vi "Calculate_duty_cycle.vi"(10 "Odour bottles in":T2(array[cluster])=[[{"Mixture components"=[{"Name"="MINERAL OIL", "CID"=0, "Volatility"=0.0}], "Name"="B1 (Bl)", "VPs"="0.0E+0", "Proportion"=[{"Numeric"=100.0}], "Selected"=FALSE, "Counter"=TRUE}, {"Mixture components"=[{"Name"="Methyl benzoate", "CID"=8103, "Volatility"=0.38}, {"Name"="Menthone", "CID"=8063, "Volatility"=0.28}], "Name"="B3 (ME2)", "VPs"="3.3E-1 ± 21%", "Proportion"=[{"Numeric"=50.0}, {"Numeric"=50.0}], "Selected"=TRUE, "Counter"=FALSE}, {"Mixture components"=[{"Name"="Decanol", "CID"=460, "Volatility"=0.00851}], "Name"="B5 (C4f)", "VPs"="8.5E-3", "Proportion"=[{"Numeric"=100.0}], "Selected"=FALSE, "Counter"=FALSE}, {"Mixture components"=[{"Name"="Acetophenone", "CID"=8174, "Volatility"=0.45}, {"Name"="Fenchone", "CID"=8635, "Volatility"=0.82}], "Name"="B7 (ME1)", "VPs"="6.4E-1 ± 41%", "Proportion"=[{"Numeric"=50.0}, {"Numeric"=50.0}], "Selected"=FALSE, "Counter"=FALSE}], [{"Mixture components"=[{"Name"="MINERAL OIL", "CID"=0, "Volatility"=0.0}], "Name"="B2 (Bl)", "VPs"="0.0E+0", "Proportion"=[{"Numeric"=100.0}], "Selected"=FALSE, "Counter"=TRUE}, {"Mixture components"=[{"Name"="Octanol", "CID"=7439, "Volatility"=0.0794}], "Name"="B4 (C4cA)", "VPs"="7.9E-2", "Proportion"=[{"Numeric"=100.0}], "Selected"=FALSE, "Counter"=FALSE}, {"Mixture components"=[{"Name"="MINERAL OIL", "CID"=0, "Volatility"=0.0}], "Name"="B6 (Bl)", "VPs"="0.0E+0", "Proportion"=[{"Numeric"=100.0}], "Selected"=FALSE, "Counter"=FALSE}, {"Mixture components"=[{"Name"="Heptanoic acid ", "CID"=957, "Volatility"=0.0107}], "Name"="B8 (C3cA)", "VPs"="1.1E-2", "Proportion"=[{"Numeric"=100.0}], "Selected"=FALSE, "Counter"=FALSE}], [{"Mixture components"=[{"Name"="MINERAL OIL", "CID"=0, "Volatility"=0.0}], "Name"="B9 (Bl)", "VPs"="0.0E+0", "Proportion"=[{"Numeric"=100.0}], "Selected"=FALSE, "Counter"=TRUE}, {"Mixture components"=[{"Name"="Geranyl acetate", "CID"=6985, "Volatility"=0.03}, {"Name"="Dimethylacetophenone", "CID"=7144, "Volatility"=0.063}], "Name"="B11 (MW1)", "VPs"="4.6E-2 ± 50%", "Proportion"=[{"Numeric"=50.0}, {"Numeric"=50.0}], "Selected"=FALSE, "Counter"=FALSE}, {"Mixture components"=[{"Name"="Geraniol", "CID"=6405, "Volatility"=0.03}, {"Name"="Phenyl butanone", "CID"=7762, "Volatility"=0.1}], "Name"="B13 (MW2)", "VPs"="6.5E-2 ± 76%", "Proportion"=[{"Numeric"=50.0}, {"Numeric"=50.0}], "Selected"=FALSE, "Counter"=FALSE}, {"Mixture components"=[{"Name"="Methylheptanoic acid", "CID"=1032, "Volatility"=0.018}], "Name"="B15 (C3f)", "VPs"="1.8E-2", "Proportion"=[{"Numeric"=100.0}], "Selected"=FALSE, "Counter"=FALSE}], [{"Mixture components"=[{"Name"="MINERAL OIL", "CID"=0, "Volatility"=0.0}], "Name"="B10 (Bl)", "VPs"="0.0E+0", "Proportion"=[{"Numeric"=100.0}], "Selected"=FALSE, "Counter"=FALSE}, {"Mixture components"=[{"Name"="Valeric acid", "CID"=8025, "Volatility"=0.196}], "Name"="B12 (C3cB)", "VPs"="2.0E-1", "Proportion"=[{"Numeric"=100.0}], "Selected"=FALSE, "Counter"=FALSE}, {"Mixture components"=[{"Name"="Nonanol", "CID"=4133, "Volatility"=0.0227}], "Name"="B14 (C4cB)", "VPs"="2.3E-2", "Proportion"=[{"Numeric"=100.0}], "Selected"=FALSE, "Counter"=FALSE}, {"Mixture components"=[{"Name"="Hydroxacetophenone", "CID"=7462, "Volatility"=0.0856}], "Name"="B16 (Ol)", "VPs"="8.6E-2", "Proportion"=[{"Numeric"=100.0}], "Selected"=FALSE, "Counter"=FALSE}]], 11 "Stimulus parameters":T1) -> (3 "Duty cycle":dbl[](array[numeric]))   [LabVIEW 2016]
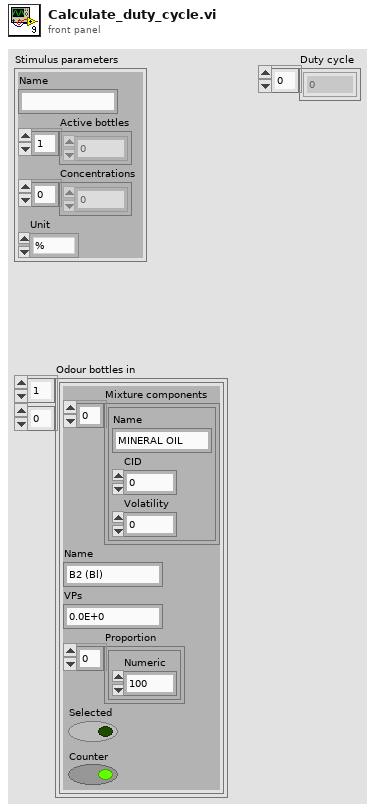
[diagram p1: front panel]
types:
  T1 = cluster{"Name":string, "Active bottles":i32[], "Concentrations":dbl[], "Unit":enum16{"%", "ppm"}}
  T2 = cluster{"Mixture components":cluster{"Name":string, "CID":i32, "Volatility":dbl}[], "Name":string, "VPs":string, "Proportion":cluster{"Numeric":dbl}[], "Selected":bool, "Counter":bool}[][]
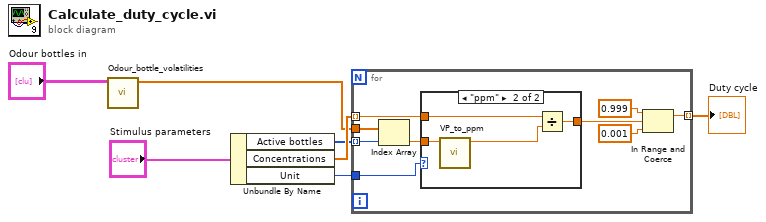
[diagram p0: block diagram]
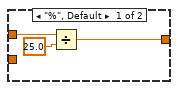
[diagram p2: hidden frame]
diagram:
  n1 = call "Odour_bottle_volatilities.vi"("Odour bottles"="Odour bottles in") -> ("Array"=w2:dbl[])  [unwired: 10 in]
  n2 = Unbundle By Name("Stimulus parameters") -> ("Active bottles"=w3:i32[], "Concentrations"=w4:dbl[], "Unit"=w5:enum16{"%", "ppm"})
  n3 = for {
    tunnel: w2 -> [w16]
    tunnel: w3 -> [w15] mode=indexing
    tunnel: w4 -> [w12] mode=indexing
    tunnel: w5 -> [w14]
    tunnel: [w8] -> w6 mode=indexing
    n4 = Index Array(array=w16, index=w15) -> (element=w13:dbl)
    n5 = case shown="\"ppm\"" w14 {
      tunnel: w13 -> [_ w23]
      tunnel: w12 -> [w19 w21]
      tunnel: [w17 w20] -> w11
      frame "%", Default {
        n6 = Divide(x=w19, y=25.0) -> (x/y=w17:dbl)
      }
      frame "ppm" {
        n7 = call "VP_to_ppm.vi"("VP (Hgmm)"=w23) -> ("Saturated concentration (ppm)"=w22:dbl)  [unwired: 10 in]
        n8 = Divide(x=w21, y=w22) -> (x/y=w20:dbl)
      }
    }
    n9 = In Range and Coerce(upper limit=0.999, x=w11, lower limit=0.001) -> (coerced(x)=w8:dbl)  [unwired: 1 out]
  }
  "Duty cycle" <- w6
